vi "Read Cursor.vi"(8 "error in (no error)":errorcluster, 11 "ControlDragSourceUpdateMsg in":refnum<class "ControlDragSourceUpdateMsg.lvclass">) -> (0 "error out":errorcluster, 2 "Cursor":refnum<k1>, 3 "ControlDragSourceUpdateMsg out":refnum<class "ControlDragSourceUpdateMsg.lvclass">)   [LabVIEW 2020, in "MVA Framework.lvlib" / "ActorEvents.lvlib" / "ControlDragSourceUpdateMsg.lvclass"]
uses:
  ControlDragSourceUpdateMsg.lvclass
  EventDataMessage/EventDataMessage.lvclass/EventDataMessage.ctl
  ControlDragSourceUpdateMsg.lvclass/ControlDragSourceUpdateMsg.ctl
  EventDataMessage/EventDataMessage.lvclass
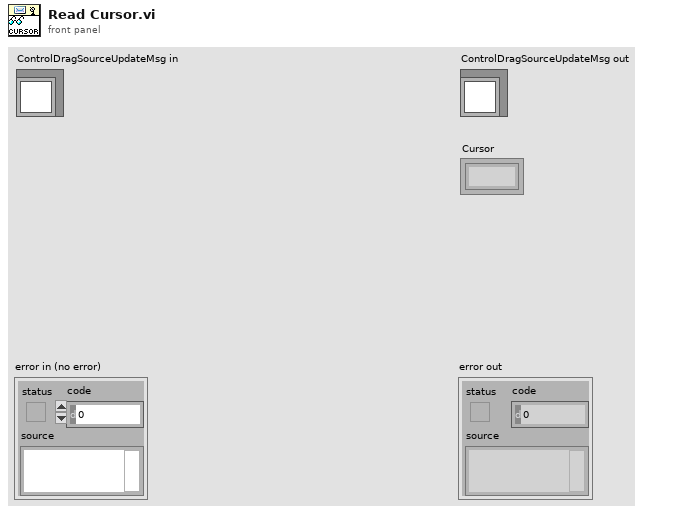
[diagram p1: front panel]
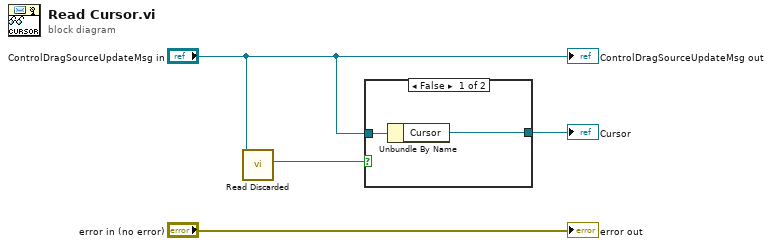
[diagram p0: block diagram]
diagram:
  n1 = call "Read Discarded.vi"("EventDataMessage in"="ControlDragSourceUpdateMsg in") -> ("Discarded?"=w2:bool)  [unwired: 8 in, 2 out]
  n2 = case shown="False" w2 {
    tunnel: [w6 _] -> w3
    tunnel: "ControlDragSourceUpdateMsg in" -> [w5 _]
    frame False {
      n3 = Unbundle By Name(w5) -> ("Cursor"=w6:refnum<k1>)
    }
    frame True {
    }
  }
  "Cursor" <- w3
  "error out" <- "error in (no error)"
  "ControlDragSourceUpdateMsg out" <- "ControlDragSourceUpdateMsg in"
